vi "力特性测试 自动对中测试.vi"(8 "error in (no error)":errorcluster caption="错误输入（无错误）") -> (0 "error out":errorcluster caption="错误输出")   [LabVIEW 2015]
doc: "该连续测量范例项目在队列消息处理器模板的基础上实现。\n\n事件处理循环负责按用户界面操作生成对应的消息。\n\n消息处理循环负责对事件处理循环或其他消息生成的消息进行处理。其中还包括用于采集和记录消息处理循环的子VI，以及用于更新图表的循环。"
uses:
  Settings/Settings.ctl
  Acquisition/Hardware Configuration.ctl
  Logging/Logging Configuration.ctl
  Motor Control/Hardware Configuration.ctl
  controls/UI Data.ctl
  controls/UI State.ctl
  Measure Type.ctl
  support/Message Queue/Enqueue Message (Single).vi
  <vilib>/Utility/error.llb/Error Cluster From Error Code.vi
  <vilib>/ErrorRing/Error Ring.xnode
  Acquisition/Acquisition.lvlib
  Logging/Logging.lvlib
  Settings/Settings.lvlib
  support/User Event - Stop/User Event - Stop.lvlib
  support/Message Queue/Message Queue.lvlib
  Motor Control/Motor Control.lvlib
panel:
  out "XY Graph":cluster{"Y":dbl[], "Y":dbl[]}[](graph) caption="扭矩VS油压"
  out "XY Graph 2":cluster{"Y":dbl[], "Y":dbl[]}[](graph) caption="角度VS油压"
  out "XY Graph 3":cluster{"Y":dbl[], "Y":dbl[]}[](graph) caption="角度VS扭矩"
  in  "转动":bool
  in  "转动角度":i32
  in  "发送按钮":bool
  in  "输入命令":string
  in  "清零":bool
  in  "读取":bool
  out "模拟通道5":dbl
  out "流量":dbl
  out "右推力":dbl
  out "左推力":dbl
  out "油压":dbl
  out "扭矩":dbl
  out "角度":dbl
  in  "计算":bool
  in  "Start":bool caption="开始"
  in  "Stop":bool caption="停止"
  out "Status":string caption="状态"
  in  "Exit":bool caption="退出"
  # "力特性测试"
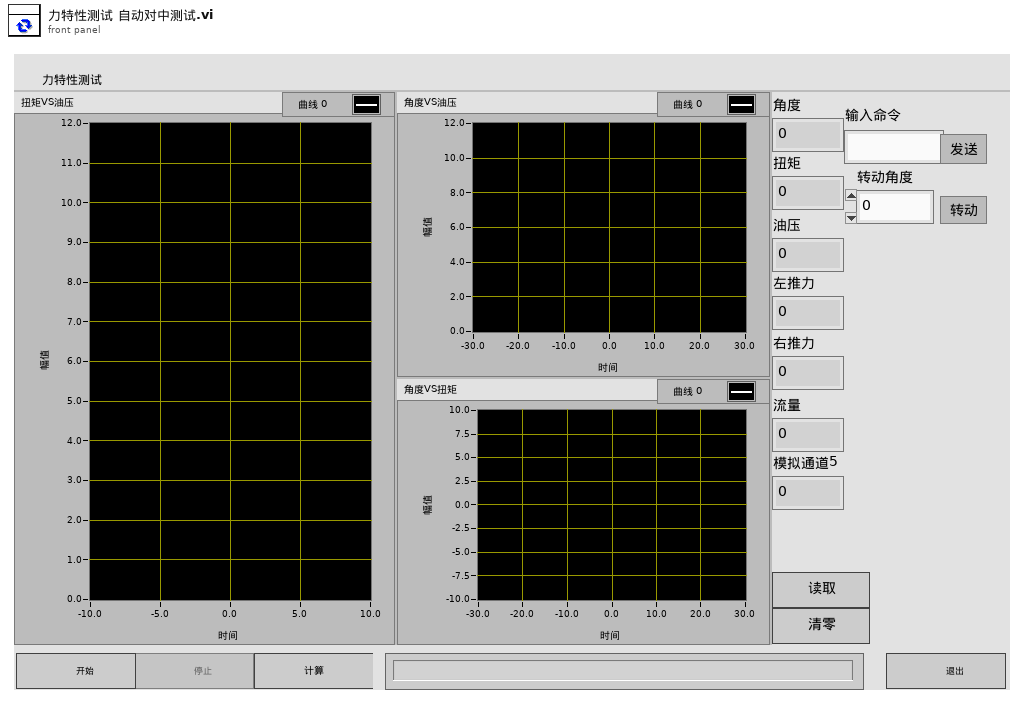
[diagram p1: front panel]
types:
  T1 = typedef "Motor Control.lvlib/电机转动逻辑1.ctl" = cluster{"反转判断条件1":T2, "停止判断条件1":T3}
  T2 = typedef "Motor Control.lvlib/反转判断条件1.ctl" = cluster{"传感器序号":i32, "条件":enum16{"小于", "大于", "等于"}, "值":dbl, "条件判断时间间隔":i32}
  T3 = typedef "Motor Control.lvlib/停止判断条件1.ctl" = cluster{"角度传感器序号":i32, "正转/反转":enum16{"正转", "反转"}, "反转次数":i32, "停止角度":dbl, "停止角度误差范围":dbl}
  T4 = typedef "UI State.ctl" = enum16{"Idle", "Acquiring and Logging", "Waiting for Exit", "Waiting for Exit (Acq Stopped)", "Waiting for Exit (Log Stopped)", "Waiting for Stop", "Waiting for Stop (Acq Stopped)", "Waiting for Stop (Log Stopped)"}
  T5 = typedef "UI Data.ctl" = cluster{"Start Ref":refnum<vi>, "Stop Ref":refnum<vi>, "calculate Ref":refnum<vi>, "Status Ref":refnum<vi>, "Exit Ref":refnum<vi>, "read Ref":refnum<vi>, "clean Ref":refnum<vi>}
  T6 = typedef "Settings.lvlib/Settings.ctl" = cluster{"Hardware Configuration":T7, "Logging Configuration":T8, "电机设置":T9, "啮合测试电机转动逻辑":T1, "功能测试电机转动逻辑":T1, "力提特性电机转动逻辑":T1}
  T7 = typedef "Acquisition.lvlib/Hardware Configuration.ctl" = cluster{"电压读取设置":cluster{"DAQmx Channel":tag, "Max Input":dbl, "Min Input":dbl, "Sample Rate":dbl, "Sample Number":i32, "DAQmx Task":refnum<k21>, "device in":tag}, "角度传感器设置":cluster{"counter":tag, "units":i32, "分辨率":i32, "初始角度":dbl, "DecodingType":i32, "A相端口":tag, "B相端口":tag, "task in":refnum<k21>}}
  T8 = typedef "Logging.lvlib/Logging Configuration.ctl" = cluster{"Log File Base Path":path, "电压传感器转换率":dbl[], "电压传感器本底":dbl[]}
  T9 = typedef "Motor Control.lvlib/Hardware Configuration.ctl" = cluster{"counter":tag, "方向端口":tag, "当前方向":bool, "频率":dbl, "DAQmx Task":refnum<k21>}
  T10 = typedef "Message Queue.lvlib/All Message Queues.ctl" = cluster{"UI":refnum<queue>, "Acquisition":refnum<queue>, "Logging":refnum<queue>, "MotorCtrl":refnum<queue>, "plot logic":refnum<queue>}
  T11 = typedef "Measure Type.ctl" = enum16{"啮合", "退回", "功能", "力特性"}
  T12 = enum8{"Enabled", "Disabled", "Disabled and Grayed Out"}
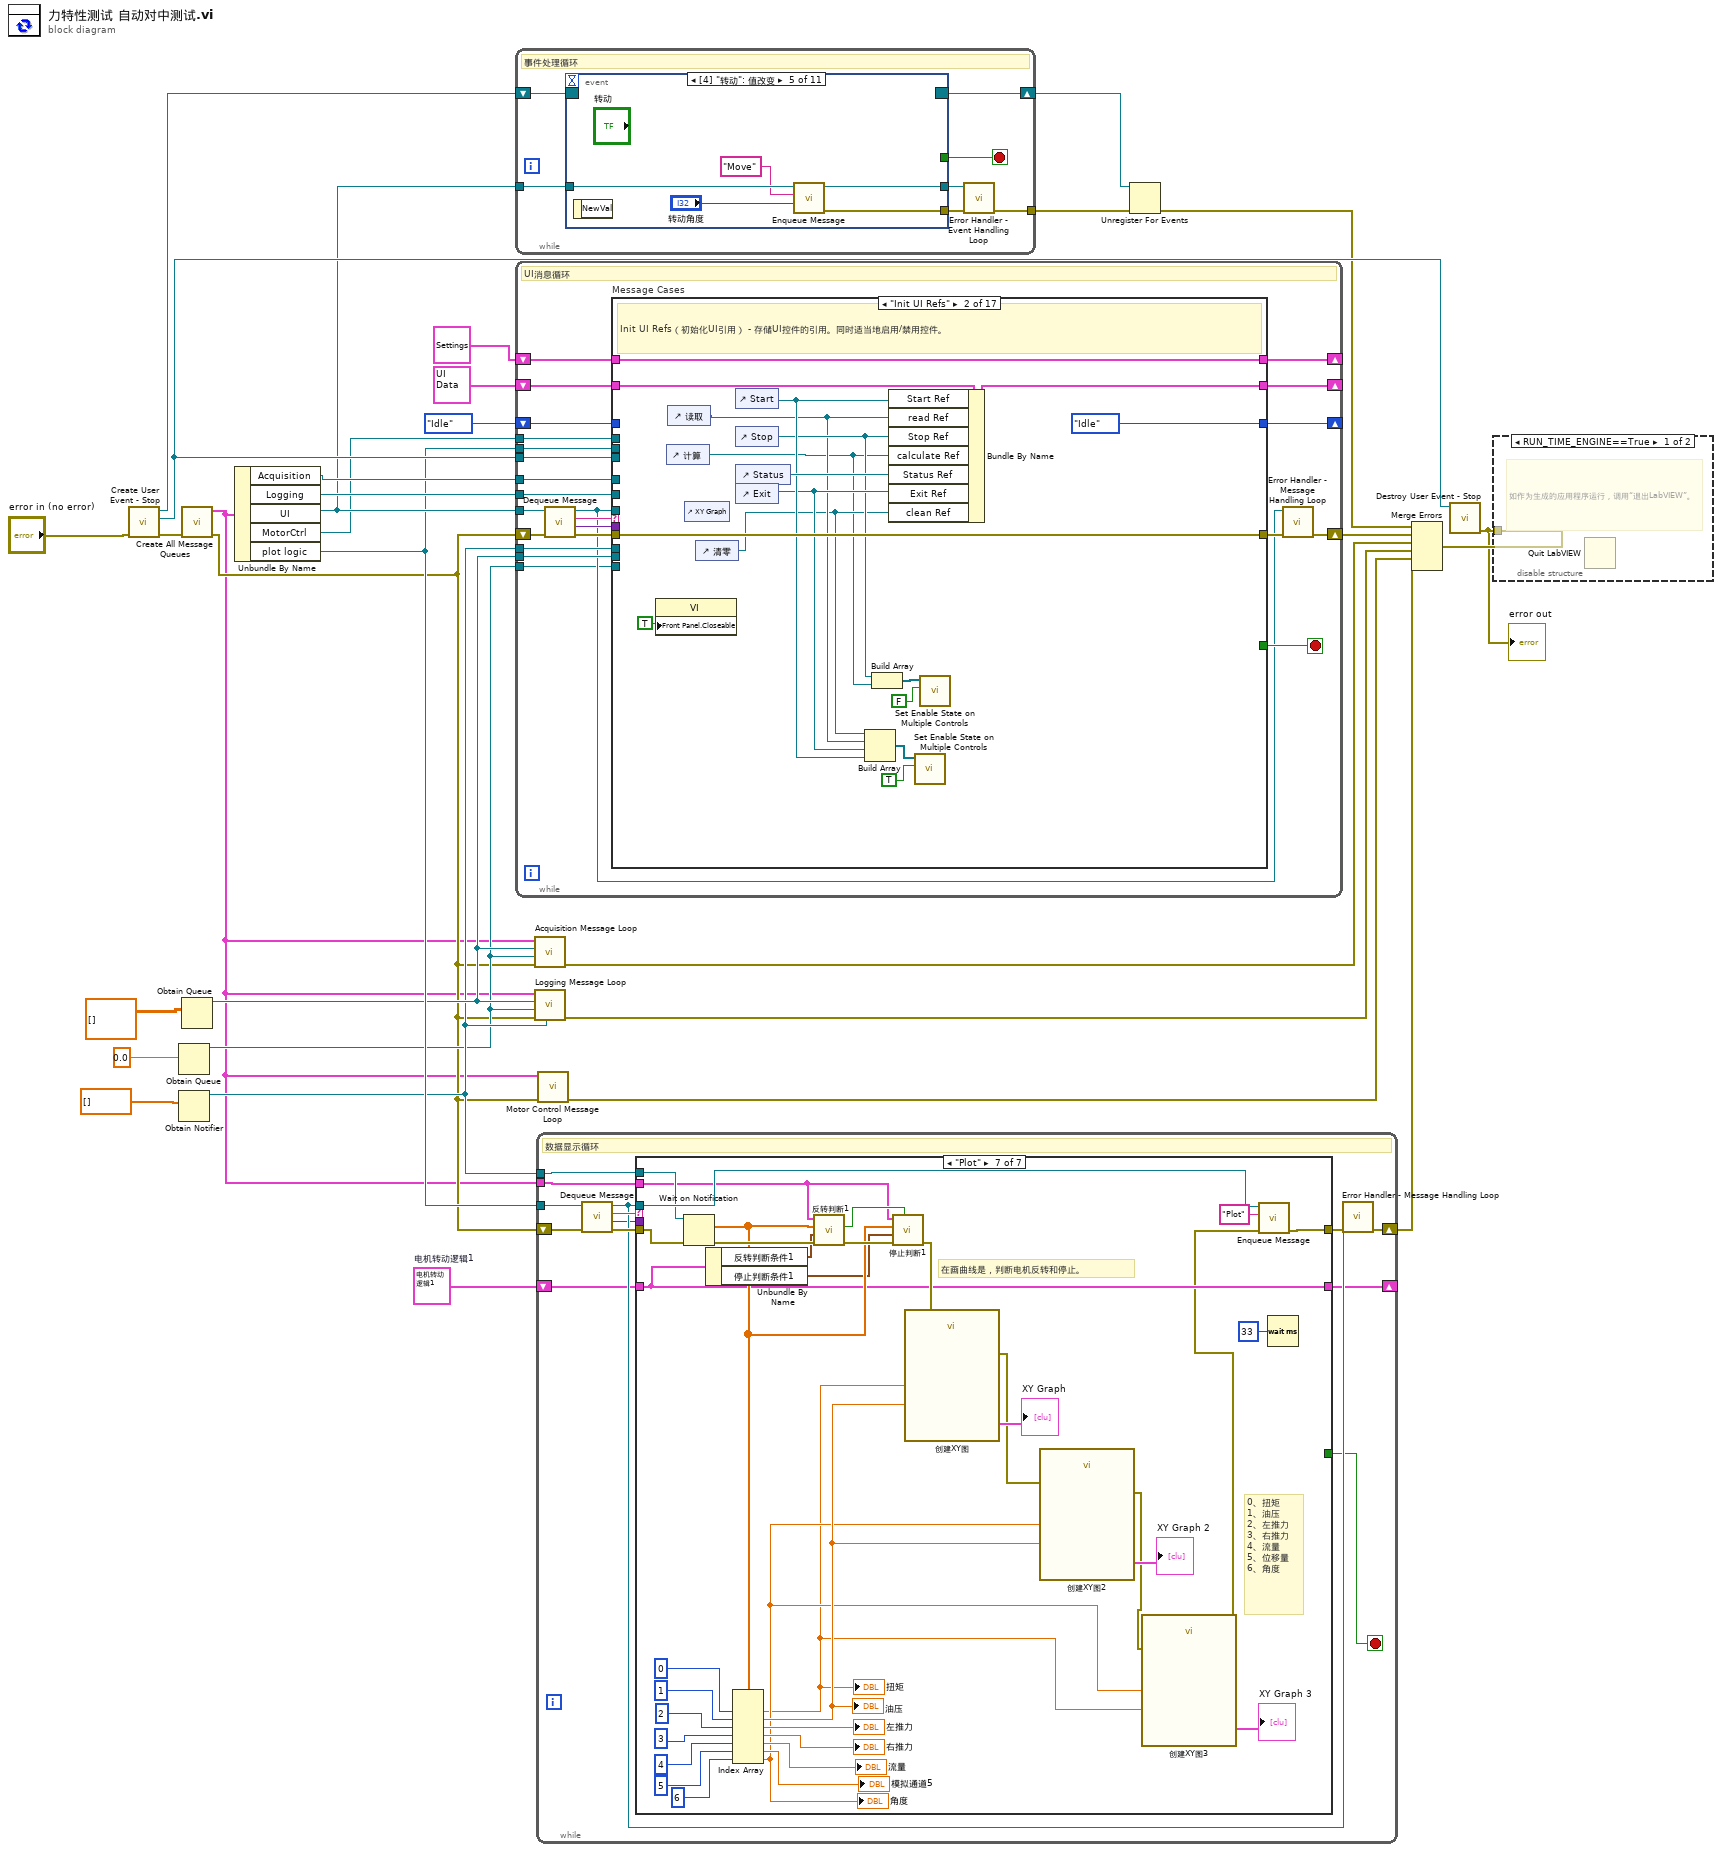
[diagram p0: block diagram]
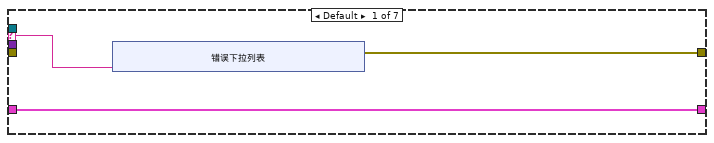
[diagram p3: hidden frame]
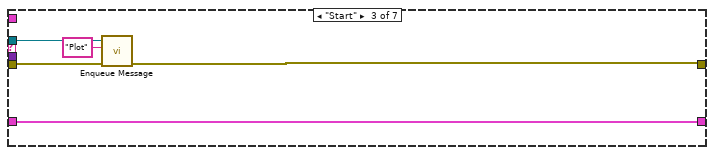
[diagram p5: hidden frame]
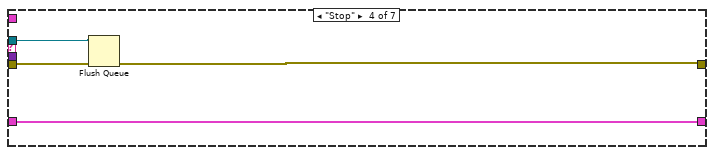
[diagram p6: hidden frame]
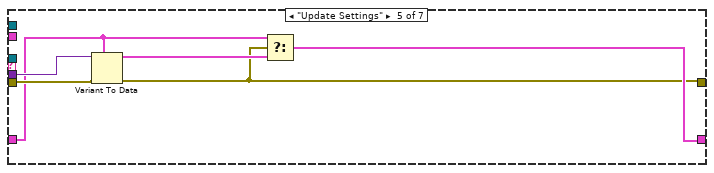
[diagram p7: hidden frame]
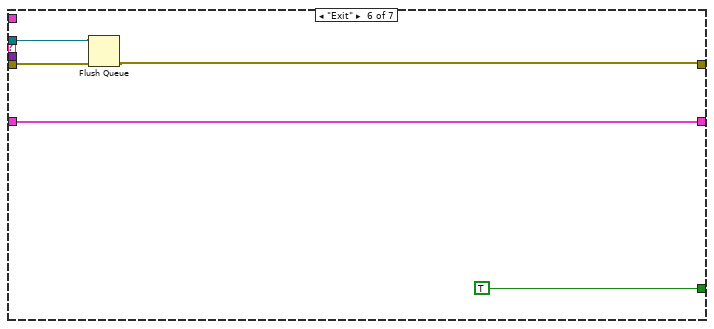
[diagram p8: hidden frame]
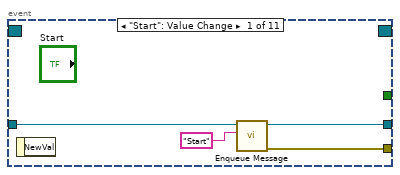
[diagram p9: hidden frame]
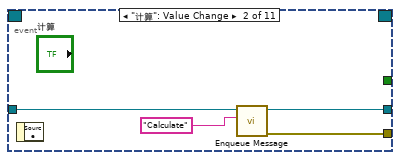
[diagram p10: hidden frame]
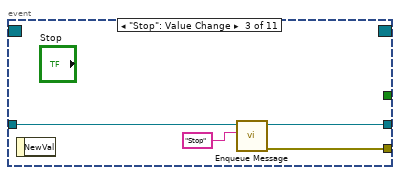
[diagram p11: hidden frame]
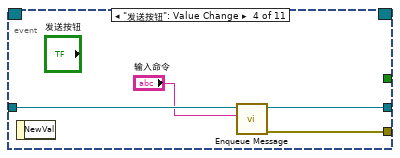
[diagram p12: hidden frame]
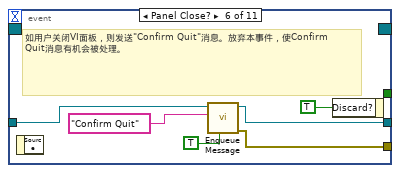
[diagram p13: hidden frame]
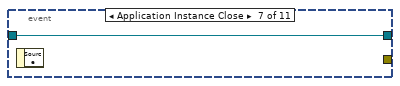
[diagram p14: hidden frame]
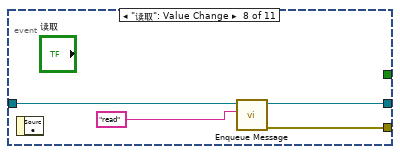
[diagram p15: hidden frame]
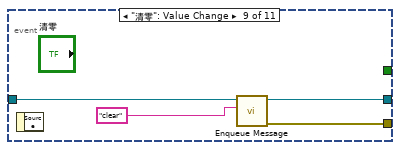
[diagram p16: hidden frame]
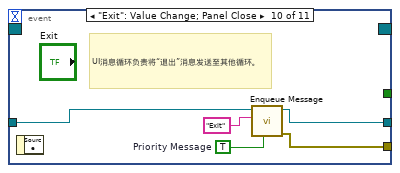
[diagram p17: hidden frame]
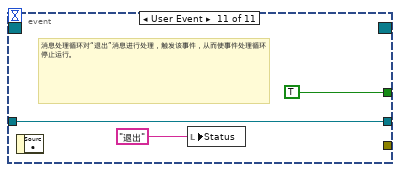
[diagram p18: hidden frame]
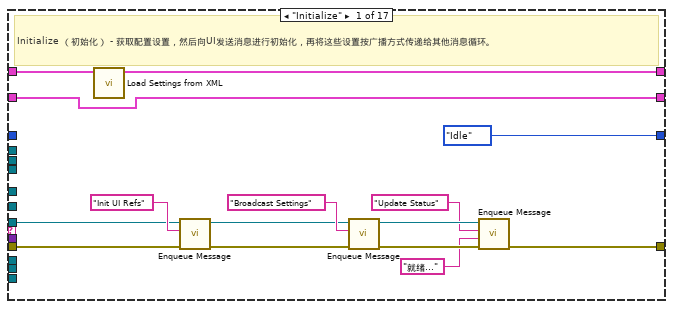
[diagram p19: hidden frame]
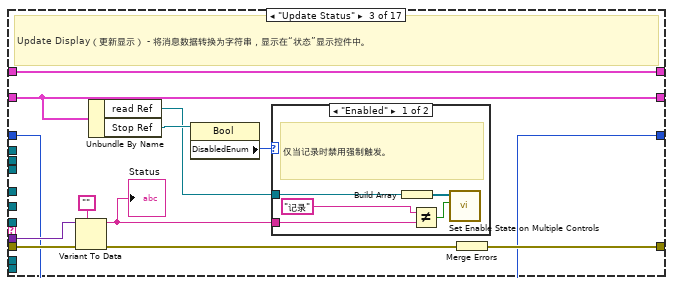
[diagram p20: hidden frame]
diagram:
  w3 = T1 {"反转判断条件1"={"传感器序号"=0, "条件"=enum."小于", "值"=0.0, "条件判断时间间隔"=0}, "停止判断条件1"={"角度传感器序号"=0, "正转/反转"=enum."正转", "反转次数"=0, "停止角度"=0.0, "停止角度误差范围"=0.0}}  # 电机转动逻辑1
  n1 = call "Create User Event - Stop.vi"("error in (no error)"="error in (no error)") -> ("error out"=w25:errorcluster, "User Event - Stop"=w27:refnum<user-event>, "Stop Event Registration Refnum"=w28:refnum<event-registration>)  [unwired: 8 in]
  n2 = Obtain Queue(element data type=0.0) -> (queue out=w8:refnum<queue>)  [unwired: 4 in, 2 out]
  n3 = Obtain Notifier(notification data type=dbl[] []) -> (notifier out=w10:refnum<notifier>)  [unwired: 3 in, 2 out]
  n4 = call "Create All Message Queues.vi"("error in (no error)"=w25) -> ("error out"=w7:errorcluster, "Message Queues out"=w4:T10)  [unwired: 9 in]
  n5 = Obtain Queue(element data type=dbl[][] []) -> (queue out=w11:refnum<queue>)  [unwired: 4 in, 2 out]
  n6 = Unbundle By Name(w4) -> ("Acquisition"=w19:refnum<queue>, "Logging"=w18:refnum<queue>, "UI"=w17:refnum<queue>, "MotorCtrl"=w15:refnum<queue>, "plot logic"=w14:refnum<queue>)
  n7 = while {
    tunnel: w17 -> [w37]
    tunnel: [w32] -> w30
    shift-right: [w36] -> w21
    shift-left: w28 -> [w38]
    stop <- w35 stop-if-true
    # "事件处理循环"
    n8 = event shown="[4] \"转动\": 值改变" {
      selector: w38 -> [_ _ _ _ _ _ _ _ _ _ _]
      dyn-events: [_ _ _ _ _ _ _ _ _ _ _] -> w36
      timeout: _ -> [_ _ _ _ _ _ _ _ _ _ _]
      tunnel: [_ _ _ _ _ _ _ _ _ _ TRUE ("Discard?")] -> w35
      tunnel: w37 -> [w40 w45 w49 w54 w59 w65 w66 w68 w72 w76 w80]
      tunnel: [w42 w44 w48 w53 w58 w60 _ w70 w74 w79 _] -> w33
      tunnel: [w39 w43 w47 w52 w57 w61 w66 w67 w71 w75 w80] -> w34
      event "Start": Value Change {
        n9 = event-data() -> ()  [unwired: 1 in, 1 out]
        n10 = call-poly "Enqueue Message.vi"("Message"="Start", "Message Queue"=w40) -> ("error out"=w42:errorcluster, "dup Message Queue"=w39:refnum<queue>)  [unwired: 8 in]
      }
      event "计算": Value Change {
        n11 = event-data() -> ()  [unwired: 1 in, 1 out]
        n12 = call-poly "Enqueue Message.vi"("Message"="Calculate", "Message Queue"=w45) -> ("error out"=w44:errorcluster, "dup Message Queue"=w43:refnum<queue>)  [unwired: 8 in]
      }
      event "Stop": Value Change {
        n13 = event-data() -> ()  [unwired: 1 in, 1 out]
        n14 = call-poly "Enqueue Message.vi"("Message"="Stop", "Message Queue"=w49) -> ("error out"=w48:errorcluster, "dup Message Queue"=w47:refnum<queue>)  [unwired: 8 in]
      }
      event "发送按钮": Value Change {
        n15 = event-data() -> ()  [unwired: 1 in, 1 out]
        n16 = call-poly "Enqueue Message.vi"("Message"="输入命令", "Message Queue"=w54) -> ("error out"=w53:errorcluster, "dup Message Queue"=w52:refnum<queue>)  [unwired: 8 in]
      }
      event "转动": Value Change {
        n17 = event-data() -> ()  [unwired: 1 in, 1 out]
        n18 = call-poly "Enqueue Message.vi"("Message Data"="转动角度", "Message"="Move", "Message Queue"=w59) -> ("error out"=w58:errorcluster, "dup Message Queue"=w57:refnum<queue>)  [unwired: 7 in]
      }
      event Panel Close? {
        # "如用户关闭VI面板，则发送\"Confirm Quit\"消息。放弃本事件，使Confirm Quit消息有机会被处理。"
        n19 = event-data() -> ()  [unwired: 1 in, 1 out]
        n20 = call-poly "Enqueue Message.vi"("Priority Message? (F)"=TRUE, "Message"="Confirm Quit", "Message Queue"=w65) -> ("error out"=w60:errorcluster, "dup Message Queue"=w61:refnum<queue>)  [unwired: 7 in]
        n21 = event-data("Discard?"=TRUE) -> ()  [unwired: 1 in, 1 out]
      }
      event Application Instance Close {
        n22 = event-data() -> ()  [unwired: 1 in, 1 out]
      }
      event "读取": Value Change {
        n23 = event-data() -> ()  [unwired: 1 in, 1 out]
        n24 = call-poly "Enqueue Message.vi"("Message"="read", "Message Queue"=w68) -> ("error out"=w70:errorcluster, "dup Message Queue"=w67:refnum<queue>)  [unwired: 8 in]
      }
      event "清零": Value Change {
        n25 = event-data() -> ()  [unwired: 1 in, 1 out]
        n26 = call-poly "Enqueue Message.vi"("Message"="clear", "Message Queue"=w72) -> ("error out"=w74:errorcluster, "dup Message Queue"=w71:refnum<queue>)  [unwired: 8 in]
      }
      event "Exit": Value Change; Panel Close {
        w77 = TRUE  # Priority Message
        # "UI消息循环负责将“退出”消息发送至其他循环。"
        n27 = event-data() -> ()  [unwired: 1 in, 1 out]
        n28 = call-poly "Enqueue Message.vi"("Priority Message? (F)"=w77, "Message"="Exit", "Message Queue"=w76) -> ("error out"=w79:errorcluster, "dup Message Queue"=w75:refnum<queue>)  [unwired: 7 in]
      }
      event User Event {
        # "消息处理循环对“退出”消息进行处理，触发该事件，从而使事件处理循环停止运行。"
        n29 = event-data() -> ()  [unwired: 1 in, 1 out]
        n30 = local write "Status"("退出" ("Exit String")) -> ()
      }
    }
    n31 = call "Error Handler - Event Handling Loop.vi"("error in (no error)"=w33, "Message Queue"=w34) -> ("dup error in"=w32:errorcluster)  [unwired: 8 in, 1 out]
  }
  n32 = while {
    tunnel: w17 -> [w99]
    tunnel: w27 -> [w104]
    shift-right: [w89] -> w31
    shift-left: w7 -> [w103]
    shift-right: [w98] -> _
    shift-left: T6 {"Hardware Configuration"={"电压读取设置"={"DAQmx Channel"="", "Max Input"=0.0, "Min Input"=0.0, "Sample Rate"=0.0, "Sample Number"=0, "DAQmx Task"="", "device in"=""}, "角度传感器设置"={"counter"="Dev1/ctr0", "units"=10146, "分辨率"=0, "初始角度"=0.0, "DecodingType"=10092, "A相端口"="/Dev1/PFI8", "B相端口"="/Dev1/PFI8", "task in"=""}}, "Logging Configuration"={"Log File Base Path"=path "", "电压传感器转换率"=[], "电压传感器本底"=[]}, "电机设置"={"counter"="Dev1/ctr0", "方向端口"="", "当前方向"=FALSE, "频率"=0.0, "DAQmx Task"=""}, "啮合测试电机转动逻辑"={"反转判断条件1"={"传感器序号"=0, "条件"=enum."小于", "值"=0.0, "条件判断时间间隔"=0}, "停止判断条件1"={"角度传感器序号"=0, "正转/反转"=enum."正转", "反转次数"=0, "停止角度"=0.0, "停止角度误差范围"=0.0}}, "功能测试电机转动逻辑"={"反转判断条件1"={"传感器序号"=0, "条件"=enum."小于", "值"=0.0, "条件判断时间间隔"=0}, "停止判断条件1"={"角度传感器序号"=0, "正转/反转"=enum."正转", "反转次数"=0, "停止角度"=0.0, "停止角度误差范围"=0.0}}, "力提特性电机转动逻辑"={"反转判断条件1"={"传感器序号"=0, "条件"=enum."小于", "值"=0.0, "条件判断时间间隔"=0}, "停止判断条件1"={"角度传感器序号"=0, "正转/反转"=enum."正转", "反转次数"=0, "停止角度"=0.0, "停止角度误差范围"=0.0}}} ("Settings") -> [w97]
    shift-right: [w95] -> _
    shift-left: T5 {"Start Ref"=refnum, "Stop Ref"=refnum, "calculate Ref"=refnum, "Status Ref"=refnum, "Exit Ref"=refnum, "read Ref"=refnum, "clean Ref"=refnum} ("Measurement UI Controls") -> [w96]
    tunnel: w19 -> [w94]
    tunnel: w18 -> [w93]
    tunnel: w10 -> [w92]
    tunnel: w11 -> [w91]
    shift-right: [w86] -> _
    shift-left: UI_State."Idle" ("UI State") -> [w87]
    tunnel: w15 -> [w83]
    tunnel: w14 -> [w84]
    tunnel: w8 -> [w85]
    stop <- w105 stop-if-true
    # "UI消息循环"
    n33 = call "Dequeue Message.vi"("error in (no error)"=w103, "Message Queue"=w99) -> ("error out"=w102:errorcluster, "Message Data"=w100:variant, "Message"=w101:string, "dup Message Queue"=w88:refnum<queue>)  [unwired: 6 in]
    n34 = case "Message Cases" shown="\"Init UI Refs\"" w101 {
      selector: w101 -> [_ _ _ _ _ _ _ _ _ _ _ _ _ _ _ _ w411]
      tunnel: w88 -> [w110 _ _ w184 _ w224 w228 w253 _ w301 w316 w326 w364 _ _ _ _]
      tunnel: w102 -> [w109 w137 w148 w183 w190 w223 w230 w255 w278 w303 w320 w325 w371 w378 w389 w405 _]
      tunnel: [w116 w137 w149 w185 w193 w225 w229 w254 w295 w298 w311 w324 w372 w377 w393 w409 w412] -> w90
      tunnel: [_ _ _ _ _ _ _ _ _ _ _ _ TRUE _ _ _ _] -> w105
      tunnel: w100 -> [_ _ w147 _ _ _ _ _ _ _ w319 _ _ _ w388 _ _]
      tunnel: w104 -> [_ _ _ _ _ _ _ _ _ _ _ _ w370 _ _ _ _]
      tunnel: [w119 w136 w144 w182 w192 w222 w234 w259 w293 w300 w322 w329 w368 w376 w392 w408 w414] -> w98
      tunnel: w97 -> [w120 w136 w144 w182 w192 w222 w234 w259 w293 w304 w322 w329 w368 w376 w392 w408 w414]
      tunnel: w96 -> [w112 w135 w143 w179 w191 w219 w233 w258 w290 w297 w321 w328 w367 w375 w391 w407 w413]
      tunnel: [w112 w134 w143 w179 w191 w219 w233 w258 w290 w297 w321 w328 w367 w375 w391 w407 w413] -> w95
      tunnel: w94 -> [_ _ _ w167 _ w207 _ _ w289 _ _ _ w366 _ _ _ _]
      tunnel: w93 -> [_ _ _ w169 w187 w210 _ _ w288 _ _ _ w365 _ _ w403 _]
      tunnel: w92 -> [_ _ _ _ _ _ _ _ _ _ _ _ w363 _ _ _ _]
      tunnel: w91 -> [_ _ _ _ _ _ _ _ _ _ _ _ w360 _ _ _ _]
      tunnel: w87 -> [_ _ w138 _ w186 w205 w232 w257 w287 w296 w310 w327 _ w374 w390 w406 w410]
      tunnel: [UI_State."Idle" ("UI State") UI_State."Idle" ("UI State") w138 UI_State."Acquiring and Logging" ("UI State") w186 w204 w231 w256 w287 w296 w310 w323 UI_State."Idle" ("UI State") w374 w390 w406 w410] -> w86
      tunnel: w85 -> [_ _ _ _ _ _ _ _ _ _ _ _ w355 _ _ _ _]
      tunnel: w84 -> [_ _ _ w161 _ w197 _ _ w282 _ _ _ w354 _ _ _ _]
      tunnel: w83 -> [_ _ _ w157 _ w195 _ _ w285 _ _ _ w353 _ w383 _ _]
      frame "Initialize" {
        # "Initialize （初始化） - 获取配置设置，然后向UI发送消息进行初始化，再将这些设置按广播方式传递给其他消息循环。"
        n35 = call "Load Settings from XML.vi"("Settings in"=w120) -> ("Settings out"=w119:T6)  [unwired: 9 in, 1 out]
        n36 = call-poly "Enqueue Message.vi"("error in (no error)"=w109, "Message"="Init UI Refs", "Message Queue"=w110) -> ("error out"=w107:errorcluster, "dup Message Queue"=w108:refnum<queue>)  [unwired: 7 in]
        n37 = call-poly "Enqueue Message.vi"("error in (no error)"=w107, "Message"="Broadcast Settings", "Message Queue"=w108) -> ("error out"=w118:errorcluster, "dup Message Queue"=w117:refnum<queue>)  [unwired: 7 in]
        n38 = call-poly "Enqueue Message.vi"("error in (no error)"=w118, "Message Data"="就绪..." ("Ready..."), "Message"="Update Status", "Message Queue"=w117) -> ("error out"=w116:errorcluster)  [unwired: 6 in, 1 out]
      }
      frame "Init UI Refs" {
        # "Init UI Refs（初始化UI引用） - 存储UI控件的引用。同时适当地启用/禁用控件。"
        n39 = property class="VI"("Front Panel.Closeable"=TRUE ("Front Panel Window:Closeable")) -> ()  [unwired: 2 in, 2 out]
        n40 = control-ref of="计算"() -> (w121:refnum<vi>)
        n41 = control-ref of="读取"() -> (w123:refnum<vi>)
        n42 = control-ref of="XY Graph"() -> ()  [unwired: 1 out]
        n43 = control-ref of="清零"() -> (w122:refnum<vi>)
        n44 = control-ref of="Start"() -> (w130:refnum<vi>)
        n45 = control-ref of="Stop"() -> (w126:refnum<vi>)
        n46 = control-ref of="Status"() -> (w131:refnum<vi>)
        n47 = control-ref of="Exit"() -> (w127:refnum<vi>)
        n48 = Build Array(w122, w123, w127, w130) -> (w129:refnum<vi>[])
        n49 = Build Array(w126, w121) -> (w125:refnum<vi>[])
        n50 = Bundle By Name(cluster=w135, "Start Ref"=w130, "read Ref"=w123, "Stop Ref"=w126, "calculate Ref"=w121, "Status Ref"=w131, "Exit Ref"=w127, "clean Ref"=w122) -> (w134:T5)
        n51 = call "Set Enable State on Multiple Controls.vi"("Enable?"=TRUE, "Controls"=w129) -> ()  [unwired: 10 in]
        n52 = call "Set Enable State on Multiple Controls.vi"("Enable?"=FALSE, "Controls"=w125) -> ()  [unwired: 10 in]
      }
      frame "Update Status" {
        # "Update Display（更新显示） - 将消息数据转换为字符串，显示在“状态”显示控件中。"
        n53 = Variant To Data(error in=w148, type="", Variant=w147) -> (data=w140:string, error out=w145:errorcluster)
        "Status" <- w140
        n54 = Unbundle By Name(w143) -> ("read Ref"=w139:refnum<vi>, "Stop Ref"=w142:refnum<vi>)
        n55 = property class="Bool"(reference=w142) -> ("DisabledEnum"=w141:T12)  [unwired: 1 in, 2 out]
        n56 = case shown="\"Enabled\"" w141 {
          tunnel: w140 -> [w152 _]
          tunnel: w139 -> [w153 _]
          frame "Enabled" {
            # "仅当记录时禁用强制触发。"
            n57 = Build Array(w153) -> (w154:refnum<vi>[])
            n58 = Not Equal?(x="记录" ("Logging"), y=w152) -> (x != y?=w150:bool)
            n59 = call "Set Enable State on Multiple Controls.vi"("Enable?"=w150, "Controls"=w154) -> ()  [unwired: 10 in]
          }
          frame "Disabled", Default {
          }
        }
        n60 = Merge Errors(w145) -> (w149:errorcluster)
      }
      frame "Start" {
        # "启用：停止\n禁用：开始、退出、设置"
        # "Start（开始） - 对于已经开始的采集，启用/禁用各个按钮并更新状态显示。"
        n61 = Unbundle By Name(w179) -> ("Stop Ref"=w162:refnum<vi>, "clean Ref"=w163:refnum<vi>, "read Ref"=w164:refnum<vi>, "Start Ref"=w174:refnum<vi>, "Exit Ref"=w173:refnum<vi>, "calculate Ref"=w172:refnum<vi>)
        n62 = call-poly "Enqueue Message.vi"("error in (no error)"=w183, "Message Data"="开始" ("Waiting for trigger"), "Message"="Update Status", "Message Queue"=w184) -> ("error out"=w171:errorcluster)  [unwired: 6 in, 1 out]
        n63 = Build Array(w162) -> (w176:refnum<vi>[])
        n64 = Build Array(w163, w164, w174, w173, w172) -> (w177:refnum<vi>[])
        n65 = call-poly "Enqueue Message.vi"("error in (no error)"=w171, "Message"="Start", "Message Queue"=w169) -> ("error out"=w168:errorcluster)  [unwired: 7 in, 1 out]
        n66 = call "Set Enable State on Multiple Controls.vi"("Enable?"=TRUE, "Controls"=w176) -> ()  [unwired: 10 in]
        n67 = call "Set Enable State on Multiple Controls.vi"("Enable?"=FALSE, "Controls"=w177) -> ()  [unwired: 10 in]
        n68 = call-poly "Enqueue Message.vi"("error in (no error)"=w168, "Message"="Start", "Message Queue"=w167) -> ("error out"=w159:errorcluster)  [unwired: 7 in, 1 out]
        n69 = call-poly "Enqueue Message.vi"("error in (no error)"=w159, "Message"="Start", "Message Queue"=w161) -> ("error out"=w158:errorcluster)  [unwired: 7 in, 1 out]
        n70 = call-poly "Enqueue Message.vi"("error in (no error)"=w158, "Message"="Start", "Message Queue"=w157) -> ("error out"=w155:errorcluster)  [unwired: 7 in, 1 out]
        n71 = Merge Errors(w155) -> (w185:errorcluster)
      }
      frame "Force Trigger" {
        # "Force Trigger（强制触发） - 发送消息至记录消息循环，开始记录。"
        n72 = call-poly "Enqueue Message.vi"("error in (no error)"=w190, "Message"="Force Trigger", "Message Queue"=w187) -> ("error out"=w189:errorcluster)  [unwired: 7 in, 1 out]
        n73 = Merge Errors(w189) -> (w193:errorcluster)
      }
      frame "Stop" {
        # "停止画图、电机、记录，最后停止采集。"
        # "启用：开始、退出、设置\n禁用：停止"
        # "停止－对于已经停止的采集，启用/禁用各个按钮并更新状态显示。"
        n74 = Unbundle By Name(w219) -> ("Stop Ref"=w201:refnum<vi>, "read Ref"=w202:refnum<vi>, "clean Ref"=w203:refnum<vi>, "Start Ref"=w214:refnum<vi>, "Exit Ref"=w213:refnum<vi>, "calculate Ref"=w212:refnum<vi>)
        n75 = call-poly "Enqueue Message.vi"("error in (no error)"=w223, "Message Data"="就绪..." ("Ready..."), "Message"="Update Status", "Message Queue"=w224) -> ("error out"=w200:errorcluster)  [unwired: 6 in, 1 out]
        n76 = Build Array(w202, w203, w214, w213, w212) -> (w217:refnum<vi>[])
        n77 = Build Array(w201) -> (w216:refnum<vi>[])
        n78 = call "Set Enable State on Multiple Controls.vi"("Enable?"=TRUE, "Controls"=w217) -> ()  [unwired: 10 in]
        n79 = call "Set Enable State on Multiple Controls.vi"("Enable?"=FALSE, "Controls"=w216) -> ()  [unwired: 10 in]
        n80 = call-poly "Enqueue Message.vi"("error in (no error)"=w200, "Message"="Stop", "Message Queue"=w197) -> ("error out"=w199:errorcluster)  [unwired: 7 in, 1 out]
        n81 = call-poly "Enqueue Message.vi"("error in (no error)"=w199, "Message"="Stop", "Message Queue"=w195) -> ("error out"=w198:errorcluster)  [unwired: 7 in, 1 out]
        n82 = call-poly "Enqueue Message.vi"("error in (no error)"=w198, "Message"="Stop", "Message Queue"=w210) -> ("error out"=w209:errorcluster)  [unwired: 7 in, 1 out]
        n83 = case shown="默认" w205 {
          selector: w205 -> [_ w227]
          tunnel: [UI_State."Waiting for Stop" ("UI State") w227] -> w204
          frame Default {
          }
          frame "Waiting for Exit" {
          }
        }
        n84 = call-poly "Enqueue Message.vi"("error in (no error)"=w209, "Message"="Stop", "Message Queue"=w207) -> ("error out"=w208:errorcluster)  [unwired: 7 in, 1 out]
        n85 = Merge Errors(w208) -> (w225:errorcluster)
      }
      frame "Acquisition Stopped" {
        # "此处代码用于确定采集停止时采取何种操作。"
        n86 = case shown="\"Waiting for Stop (Log Stopped)\"" w232 {
          selector: w232 -> [w236 _ _ _ _]
          tunnel: [w236 UI_State."Waiting for Exit (Acq Stopped)" ("UI State") UI_State."Waiting for Stop (Acq Stopped)" ("UI State") UI_State."Idle" ("UI State") UI_State."Idle" ("UI State")] -> w231
          tunnel: w230 -> [w235 w237 w239 w245 w251]
          tunnel: [w235 w237 w239 w244 w250] -> w229
          tunnel: w228 -> [_ _ _ w243 w249]
          frame Default {
          }
          frame "Waiting for Exit", "Waiting for Exit (Acq Stopped)" {
          }
          frame "Waiting for Stop", "Waiting for Stop (Acq Stopped)" {
          }
          frame "Waiting for Exit (Log Stopped)" {
            # "如果正在等待退出且记录已结束，“采集停止”消息表示应退出。"
            n87 = call-poly "Enqueue Message.vi"("Priority Message? (F)"=TRUE, "error in (no error)"=w245, "Message"="Exit", "Message Queue"=w243) -> ("error out"=w244:errorcluster)  [unwired: 6 in, 1 out]
          }
          frame "Waiting for Stop (Log Stopped)" {
            # "当前状态为等待停止时，如已停止记录，则收到\"Acquisition Stopped\"消息时即可停止。"
            n88 = call-poly "Enqueue Message.vi"("error in (no error)"=w251, "Message Data"="Ready..." ("Message"), "Message"="Update Status", "Message Queue"=w249) -> ("error out"=w250:errorcluster)  [unwired: 6 in, 1 out]
          }
        }
      }
      frame "Logging Stopped" {
        # "此处代码用于确定记录停止时采取何种操作。"
        n89 = case shown="\"Waiting for Stop (Acq Stopped)\"" w257 {
          selector: w257 -> [w261 _ _ _ _]
          tunnel: [w261 UI_State."Waiting for Exit (Log Stopped)" ("UI State") UI_State."Waiting for Stop (Log Stopped)" ("UI State") UI_State."Idle" ("UI State") UI_State."Idle" ("UI State")] -> w256
          tunnel: w255 -> [w260 w262 w264 w270 w276]
          tunnel: [w260 w262 w264 w269 w275] -> w254
          tunnel: w253 -> [_ _ _ w268 w274]
          frame Default {
          }
          frame "Waiting for Exit", "Waiting for Exit (Log Stopped)" {
          }
          frame "Waiting for Stop", "Waiting for Stop (Log Stopped)" {
          }
          frame "Waiting for Exit (Acq Stopped)" {
            # "如果正在等待退出且采集已结束，“记录停止”消息表示应退出。"
            n90 = call-poly "Enqueue Message.vi"("Priority Message? (F)"=TRUE, "error in (no error)"=w270, "Message"="Exit", "Message Queue"=w268) -> ("error out"=w269:errorcluster)  [unwired: 6 in, 1 out]
          }
          frame "Waiting for Stop (Acq Stopped)" {
            # "如果正在等待停止且采集已结束，“记录停止”消息表示应停止。"
            n91 = call-poly "Enqueue Message.vi"("error in (no error)"=w276, "Message Data"="Ready..." ("Message"), "Message"="Update Status", "Message Queue"=w274) -> ("error out"=w275:errorcluster)  [unwired: 6 in, 1 out]
          }
        }
      }
      frame "Broadcast settings" {
        w281 = "Update Settings" ("Message")
        # "向“记录和采集”消息队列发送“更新设置”消息。"
        n92 = Unbundle By Name(w293) -> ("Hardware Configuration"=w292:T7, "Logging Configuration"=w291:T8, "电机设置"=w284:T9, "啮合测试电机转动逻辑"=w280:T1)
        n93 = call-poly "Enqueue Message.vi"("error in (no error)"=w278, "Message Data"=w292, "Message"=w281, "Message Queue"=w289) -> ("error out"=w294:errorcluster)  [unwired: 6 in, 1 out]
        n94 = call-poly "Enqueue Message.vi"("error in (no error)"=w294, "Message Data"=w291, "Message"=w281, "Message Queue"=w288) -> ("error out"=w286:errorcluster)  [unwired: 6 in, 1 out]
        n95 = call-poly "Enqueue Message.vi"("error in (no error)"=w286, "Message Data"=w284, "Message"=w281, "Message Queue"=w285) -> ("error out"=w283:errorcluster)  [unwired: 6 in, 1 out]
        n96 = call-poly "Enqueue Message.vi"("error in (no error)"=w283, "Message Data"=w280, "Message"=w281, "Message Queue"=w282) -> ("error out"=w279:errorcluster)  [unwired: 6 in, 1 out]
        n97 = Merge Errors(w279, w278) -> (w295:errorcluster)
      }
      frame "Launch Settings Dialog" {
        # "用户单击“设置”按钮时，启动设置对话框。"
        n98 = call "Settings Dialog.vi"("error in (no error)"=w303, "Settings in"=w304) -> ("error out"=w299:errorcluster, "Cancelled?"=w302:bool, "Settings out"=w300:T6)  [unwired: 6 in, 1 out]
        n99 = case shown="假" w302 {
          tunnel: w301 -> [w308 _]
          tunnel: w299 -> [w307 w309]
          tunnel: [w306 w309] -> w298
          frame False {
            n100 = call-poly "Enqueue Message.vi"("error in (no error)"=w307, "Message"="Broadcast Settings", "Message Queue"=w308) -> ("error out"=w306:errorcluster)  [unwired: 7 in, 1 out]
          }
          frame True {
          }
        }
      }
      frame "Error" {
        # "Error - 检查错误消息数据及其响应。该消息由应用程序各循环结束处的“错误处理”VI发送。"
        n101 = Variant To Data(error in=w320, type=errorcluster {"status"=FALSE, "code"=0, "source"=""} ("error out"), Variant=w319) -> (data=w317:errorcluster, error out=w313:errorcluster)
        n102 = call <vilib>:"Simple Error Handler.vi"("error in (no error)"=w317) -> ()  [unwired: 4 in, 5 out]
        n103 = call-poly "Enqueue Message.vi"("Priority Message? (F)"=TRUE, "Message"="Exit", "Message Queue"=w316) -> ("error out"=w312:errorcluster)  [unwired: 7 in, 1 out]
        n104 = Merge Errors(w312, w313) -> (w311:errorcluster)
      }
      frame "Confirm Quit" {
        # "Confirm Quit - 该消息用于确认用户是否需要退出应用程序。"
        n105 = case shown="\"Acquiring and Logging\"" w327 {
          tunnel: w326 -> [w334 w340]
          tunnel: w325 -> [w333 w338]
          tunnel: [w330 w337] -> w324
          tunnel: [UI_State."Idle" ("UI State") w336] -> w323
          frame Default {
            # "如收到'Confirm Quit'消息时系统处于空闲状态，则不需要弹出确认提示。"
            n106 = call-poly "Enqueue Message.vi"("Priority Message? (F)"=TRUE, "error in (no error)"=w333, "Message"="Exit", "Message Queue"=w334) -> ("error out"=w330:errorcluster)  [unwired: 6 in, 1 out]
          }
          frame "Acquiring and Logging" {
            n107 = Two Button Dialog(message="采集仍在执行中，是否确定退出？" ("Confirm Quit Message"), 1:"否" ("No"), 2:"是" ("Yes")) -> (T button?=w339:bool)
            n108 = case shown="真" w339 {
              tunnel: w340 -> [_ w350]
              tunnel: w338 -> [w344 w349]
              tunnel: [w344 w348] -> w337
              tunnel: [UI_State."Acquiring and Logging" ("UI State") UI_State."Waiting for Exit" ("UI State")] -> w336
              frame False {
                # "用户不希望退出。"
              }
              frame True {
                n109 = call-poly "Enqueue Message.vi"("error in (no error)"=w349, "Message"="Stop", "Message Queue"=w350) -> ("error out"=w348:errorcluster)  [unwired: 7 in, 1 out]
              }
            }
          }
        }
      }
      frame "Exit" {
        w351 = TRUE ("Priority Message? (F)")
        w352 = "Exit" ("Message")
        # "不必检查错误输出。采集和记录队列可能已被释放。"
        # "停止VI。"
        # "Exit（退出）－触发用户事件，使“事件处理”循环停止运行。同时向“采集和记录”循环发送“退出”消息。"
        n110 = Release Queue(queue=w364, error in (no error)=w371) -> (error out=w362:errorcluster)  [unwired: 1 in, 2 out]
        n111 = call "Fire User Event - Stop.vi"("User Event - Stop"=w370) -> ("error out"=w369:errorcluster)  [unwired: 10 in]
        n112 = Release Notifier(notifier=w363, error in (no error)=w362) -> (error out=w361:errorcluster)  [unwired: 1 in, 2 out]
        n113 = Release Queue(queue=w360, error in (no error)=w361) -> (error out=w357:errorcluster)  [unwired: 1 in, 2 out]
        n114 = call-poly "Enqueue Message.vi"("Priority Message? (F)"=TRUE, "Message"=w352, "Message Queue"=w366) -> ()  [unwired: 7 in, 2 out]
        n115 = Release Queue(queue=w355, error in (no error)=w357) -> (error out=w356:errorcluster)  [unwired: 1 in, 2 out]
        n116 = call-poly "Enqueue Message.vi"("Priority Message? (F)"=w351, "Message"=w352, "Message Queue"=w365) -> ()  [unwired: 7 in, 2 out]
        n117 = call-poly "Enqueue Message.vi"("Priority Message? (F)"=w351, "Message"=w352, "Message Queue"=w354) -> ()  [unwired: 7 in, 2 out]
        n118 = call-poly "Enqueue Message.vi"("Priority Message? (F)"=w351, "Message"=w352, "Message Queue"=w353) -> ()  [unwired: 7 in, 2 out]
        n119 = Merge Errors(w369, w356) -> (w372:errorcluster)
      }
      frame "---Copy This Frame---" {
        # "如需创建新消息，可创建该帧的副本。在副本中，将本注释更改为对应消息的注释。"
        n120 = Merge Errors(w378) -> (w377:errorcluster)
      }
      frame "Move" {
        # "角度是负数，说明需要反转，\n发送Turn指令转向。"
        # "如需创建新消息，可创建该帧的副本。在副本中，将本注释更改为对应消息的注释。"
        n121 = Variant To Data(error in=w389, type=0, Variant=w388) -> (data=w379:i32, error out=w385:errorcluster)
        n122 = Less Than 0?(x=w379) -> (x < 0?=w386:bool)
        n123 = case shown="真" w386 {
          tunnel: w385 -> [w395 w400]
          tunnel: [w395 w399] -> w384
          tunnel: w383 -> [w394 w398]
          tunnel: [w394 w396] -> w381
          frame False {
          }
          frame True {
            n124 = call-poly "Enqueue Message.vi"("error in (no error)"=w400, "Message"="Turn", "Message Queue"=w398) -> ("error out"=w399:errorcluster, "dup Message Queue"=w396:refnum<queue>)  [unwired: 7 in]
          }
        }
        n125 = call-poly "Enqueue Message.vi"("error in (no error)"=w384, "Message Data"=w379, "Message"="Move", "Message Queue"=w381) -> ("error out"=w382:errorcluster)  [unwired: 6 in, 1 out]
        n126 = Merge Errors(w382) -> (w393:errorcluster)
      }
      frame "Calculate" {
        # "发指令让记录线程执行计算，传入相应的计算类型。"
        # "如需创建新消息，可创建该帧的副本。在副本中，将本注释更改为对应消息的注释。"
        n127 = call-poly "Enqueue Message.vi"("error in (no error)"=w405, "Message Data"=Measure_Type."力特性" ("计算类型"), "Message"="Calculate", "Message Queue"=w403) -> ("error out"=w404:errorcluster)  [unwired: 6 in, 1 out]
        n128 = Merge Errors(w404) -> (w409:errorcluster)
      }
      frame Default {
        # "如得到的消息未经任何分支定义，则运行“默认”分支。输出程序错误。"
        n129 = xnode "错误下拉列表"("参数 0"=w411) -> ("错误输出"=w412:errorcluster)
      }
    }
    n130 = call "Error Handler - Message Handling Loop.vi"("error in (no error)"=w90, "Message Queue"=w88) -> ("dup error in"=w89:errorcluster)  [unwired: 8 in, 1 out]
  }
  n131 = call "Acquisition Message Loop.vi"("error in (no error)"=w7, "Angle Data Queue"=w8, "Analog Data Queue"=w11, "Message Queues"=w4) -> ("error out"=w26:errorcluster)  [unwired: 7 in]
  n132 = call "Logging Message Loop.vi"("数据通知器"=w10, "error in (no error)"=w7, "Angle Data Queue"=w8, "Analog Data Queue"=w11, "Message Queues"=w4) -> ("error out"=w24:errorcluster)  [unwired: 6 in]
  n133 = while "Data Display Loop" {
    tunnel: w10 -> [w427]
    tunnel: w14 -> [w434]
    shift-right: [w429] -> w5
    shift-left: w7 -> [w433]
    tunnel: w4 -> [w425]
    shift-right: [w422] -> _
    shift-left: w3 -> [w423]
    stop <- w426 stop-if-true
    # "数据显示循环"
    n134 = call "Dequeue Message.vi"("error in (no error)"=w433, "Message Queue"=w434) -> ("error out"=w431:errorcluster, "Message Data"=w424:variant, "Message"=w430:string, "dup Message Queue"=w428:refnum<queue>)  [unwired: 6 in]
    n135 = case shown="\"Plot\"" w430 {
      selector: w430 -> [w436 _ _ _ _ _ _]
      tunnel: [w437 w445 w448 w454 w456 w464 w485] -> w432
      tunnel: w431 -> [_ w445 w451 w455 w460 w466 w498]
      tunnel: w428 -> [_ _ w450 w453 _ w465 w501]
      tunnel: w427 -> [_ _ _ _ _ _ w499]
      tunnel: [_ _ _ _ _ TRUE _] -> w426
      tunnel: w425 -> [_ _ _ _ _ _ w481]
      tunnel: w424 -> [_ _ _ _ w459 _ _]
      tunnel: [w435 w446 w447 w452 w457 w462 w478] -> w422
      tunnel: w423 -> [w435 w446 w447 w452 w458 w462 w478]
      frame Default {
        n136 = xnode "错误下拉列表"("参数 0"=w436) -> ("错误输出"=w437:errorcluster)
      }
      frame "Initialize" {
      }
      frame "Start" {
        n137 = call-poly "Enqueue Message.vi"("error in (no error)"=w451, "Message"="Plot", "Message Queue"=w450) -> ("error out"=w448:errorcluster)  [unwired: 7 in, 1 out]
      }
      frame "Stop" {
        n138 = Flush Queue(queue=w453, error in (no error)=w455) -> (error out=w454:errorcluster)  [unwired: 2 out]
      }
      frame "Update Settings" {
        n139 = Variant To Data(error in=w460, type=w458, Variant=w459) -> (data=w461:T1, error out=w456:errorcluster)
        n140 = Select(t=w458, s=w456, f=w461) -> (s? t:f=w457:T1)
      }
      frame "Exit" {
        n141 = Flush Queue(queue=w465, error in (no error)=w466) -> (error out=w464:errorcluster)  [unwired: 2 out]
      }
      frame "Plot" {
        # "在画曲线是，判断电机反转和停止。"
        # "0、扭矩\n1、油压\n2、左推力\n3、右推力\n4、流量\n5、位移量\n6、角度"
        n142 = Wait on Notification(notifier=w499, error in (no error)=w498) -> (notification=w480:dbl[], error out=w484:errorcluster)  [unwired: 2 in, 2 out]
        n143 = Unbundle By Name(w478) -> ("反转判断条件1"=w477:T2, "停止判断条件1"=w476:T3)
        n144 = Index Array(array=w480, index #1=0 ("索引"), index #2=1 ("索引"), index #3=2 ("索引"), index #4=3 ("索引"), index #5=4 ("索引"), index #6=5 ("索引"), index #7=6 ("索引")) -> (element #1=w468:dbl, element #2=w470:dbl, element #3=→"左推力":dbl, element #4=→"右推力":dbl, element #5=→"流量":dbl, element #6=→"模拟通道5":dbl, element #7=w469:dbl)
        "角度" <- w469
        "扭矩" <- w468
        "油压" <- w470
        n145 = call "反转判断1.vi"("error in (no error)"=w484, "反转判断条件1"=w477, "传感器数据"=w480, "Message Queues"=w481) -> ("error out"=w483:errorcluster, "反转"=w482:bool)  [unwired: 6 in]
        n146 = call "停止判断1.vi"("反转？"=w482, "error in (no error)"=w483, "反转判断条件1"=w476, "传感器数据"=w480, "Message Queues"=w481) -> ("error out"=w479:errorcluster)  [unwired: 6 in]
        n147 = call "创建XY图"("error in (no error)"=w479, "Y Input"=w470, "X Input"=w468) -> ("error out"=w473:errorcluster, "XY Graph"=→"XY Graph":cluster{"X":dbl[], "Y":dbl[]}[])  [unwired: 7 in]
        n148 = call "创建XY图2"("error in (no error)"=w473, "Y Input"=w470, "X Input"=w469) -> ("error out"=w472:errorcluster, "XY Graph"=→"XY Graph 2":cluster{"X":dbl[], "Y":dbl[]}[])  [unwired: 7 in]
        n149 = call "创建XY图3"("error in (no error)"=w472, "Y Input"=w468, "X Input"=w469) -> ("error out"=w471:errorcluster, "XY Graph"=→"XY Graph 3":cluster{"X":dbl[], "Y":dbl[]}[])  [unwired: 7 in]
        n150 = call-poly "Enqueue Message.vi"("error in (no error)"=w471, "Message"="Plot", "Message Queue"=w501) -> ("error out"=w485:errorcluster)  [unwired: 7 in, 1 out]
        n151 = Wait (ms)(milliseconds to wait=u32 33 ("等待时间（毫秒）")) -> ()  [unwired: 1 out]
      }
    }
    n152 = call "Error Handler - Message Handling Loop.vi"("error in (no error)"=w432, "Message Queue"=w428) -> ("dup error in"=w429:errorcluster)  [unwired: 8 in, 1 out]
  }
  n153 = call "Motor Control Message Loop.vi"("error in (no error)"=w7, "Message Queues"=w4) -> ("error out"=w6:errorcluster)  [unwired: 9 in]
  n154 = Unregister For Events(event registration refnum=w21, error in=w30) -> (error out=w22:errorcluster)
  n155 = Merge Errors(w22, w31, w26, w24, w6, w5) -> (w29:errorcluster)
  n156 = call "Destroy User Event - Stop.vi"("error in (no error)"=w29, "User Event - Stop"=w27) -> ("error out"=w2:errorcluster)  [unwired: 9 in]
  "error out" <- w2
  n157 = disable-structure shown="RUN_TIME_ENGINE==True" {
    disable-tunnel: w2 -> [_ _]
    frame condition #0 {
      # "如作为生成的应用程序运行，调用“退出LabVIEW”。"
      n158 = Quit LabVIEW() -> ()  [unwired: 1 in]
    }
    frame condition #1 (active) {
    }
  }
